vi "Read Memory.vi"(8 "error in (no error)":errorcluster, 10 "Memory Address":i32, 11 "gScript Interpreter in":refnum<class "gScript Interpreter.lvclass">) -> (0 "error out":errorcluster, 2 "Memory Cell":T1, 3 "gScript Interpreter out":refnum<class "gScript Interpreter.lvclass">)   [LabVIEW 2017, in "gScript Interpreter.lvclass"]
uses:
  gScript Interpreter.lvclass
  Type Definitions/Memory Cell.ctl
  Type Definitions/Memory Cell Type Enum.ctl
  gScript Interpreter.lvclass/gScript Interpreter.ctl
  <vilib>/Utility/error.llb/Error Cluster From Error Code.vi
  <vilib>/ErrorRing/Error Ring.xnode
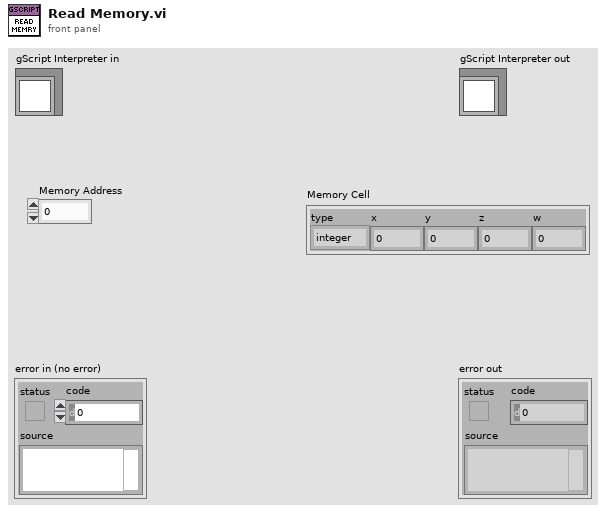
[diagram p1: front panel]
types:
  T1 = typedef "Memory Cell.ctl" = cluster{"type":T2, "x":dbl, "y":dbl, "z":dbl, "w":dbl}
  T2 = typedef "Memory Cell Type Enum.ctl" = enum16{"integer", "float", "vector", "rotation"}
  T3 = typedef "Main Memory.ctl" = T1[]
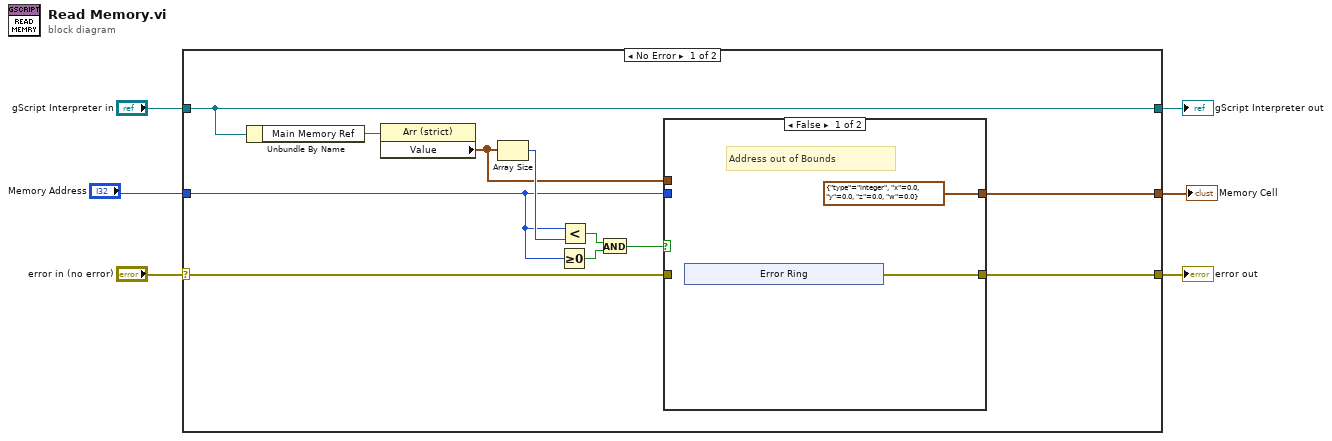
[diagram p0: block diagram]
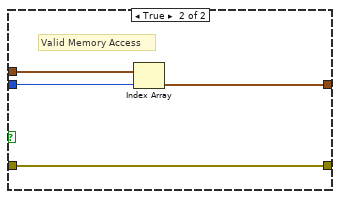
[diagram p2: hidden frame]
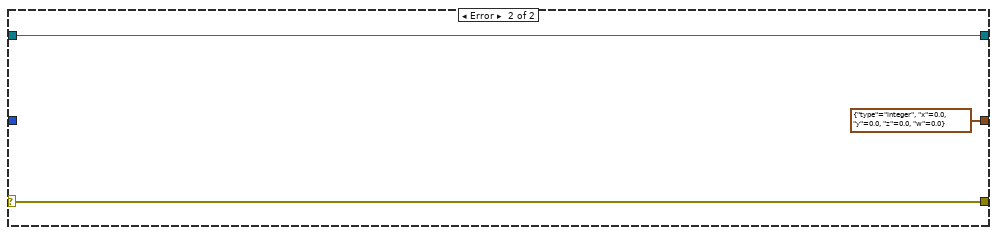
[diagram p3: hidden frame]
diagram:
  n1 = case shown="No Error" "error in (no error)" {
    selector: "error in (no error)" -> [w14 w30]
    tunnel: [w13 w30] -> w5
    tunnel: [w17 w29] -> w3
    tunnel: "gScript Interpreter in" -> [w17 w29]
    tunnel: "Memory Address" -> [w7 _]
    tunnel: [w15 T1 {"type"=enum."integer", "x"=0.0, "y"=0.0, "z"=0.0, "w"=0.0} ("Memory Cell")] -> w2
    frame No Error {
      n2 = Unbundle By Name(w17) -> ("Main Memory Ref"=w16:refnum<vi>)
      n3 = property class="Arr (strict)"(reference=w16) -> ("Value"=w8:T3)  [unwired: 1 in, 2 out]
      n4 = Array Size(array=w8) -> (size(s)=w12:i32)
      n5 = Greater Or Equal To 0?(x=w7) -> (x >= 0?=w10:bool)
      n6 = Less?(x=w7, y=w12) -> (x < y?=w11:bool)
      n7 = And(x=w11, y=w10) -> (x .and. y?=w9:bool)
      n8 = case shown="False" w9 {
        tunnel: w8 -> [_ w26]
        tunnel: [T1 {"type"=enum."integer", "x"=0.0, "y"=0.0, "z"=0.0, "w"=0.0} ("Memory Cell") w24] -> w15
        tunnel: w14 -> [_ w27]
        tunnel: [w18 w27] -> w13
        tunnel: w7 -> [_ w25]
        frame False {
          # "Address out of Bounds"
          n9 = xnode "Error Ring"() -> ("error out"=w18:errorcluster)
        }
        frame True {
          # "Valid Memory Access"
          n10 = Index Array(array=w26, index=w25) -> (element=w24:T1)
        }
      }
    }
    frame Error {
    }
  }
  "error out" <- w5
  "gScript Interpreter out" <- w3
  "Memory Cell" <- w2
